vi "Basci_VIs_FindIndexByKeyWords.vi"(4 "error in (no error)":errorcluster, 5 "Max length\nof index":i32=4, 6 "Key words":string="Trace_", 7 "String input":string) -> (0 "error out":errorcluster, 1 "Log":string, 2 "# boundaries between char and digit":i32, 3 "Folder index":i32)   [LabVIEW 2017, in "BasicVIs.lvlib"]
uses:
  BasicVIs.lvlib
panel:
  out "Numeric":i32
  out "Array":u8[](array[numeric])
  out "has digit":bool
  out "has NaN":bool
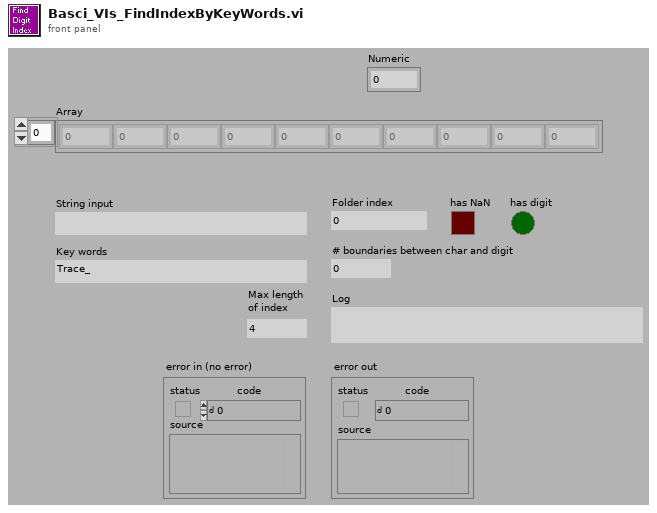
[diagram p1: front panel]
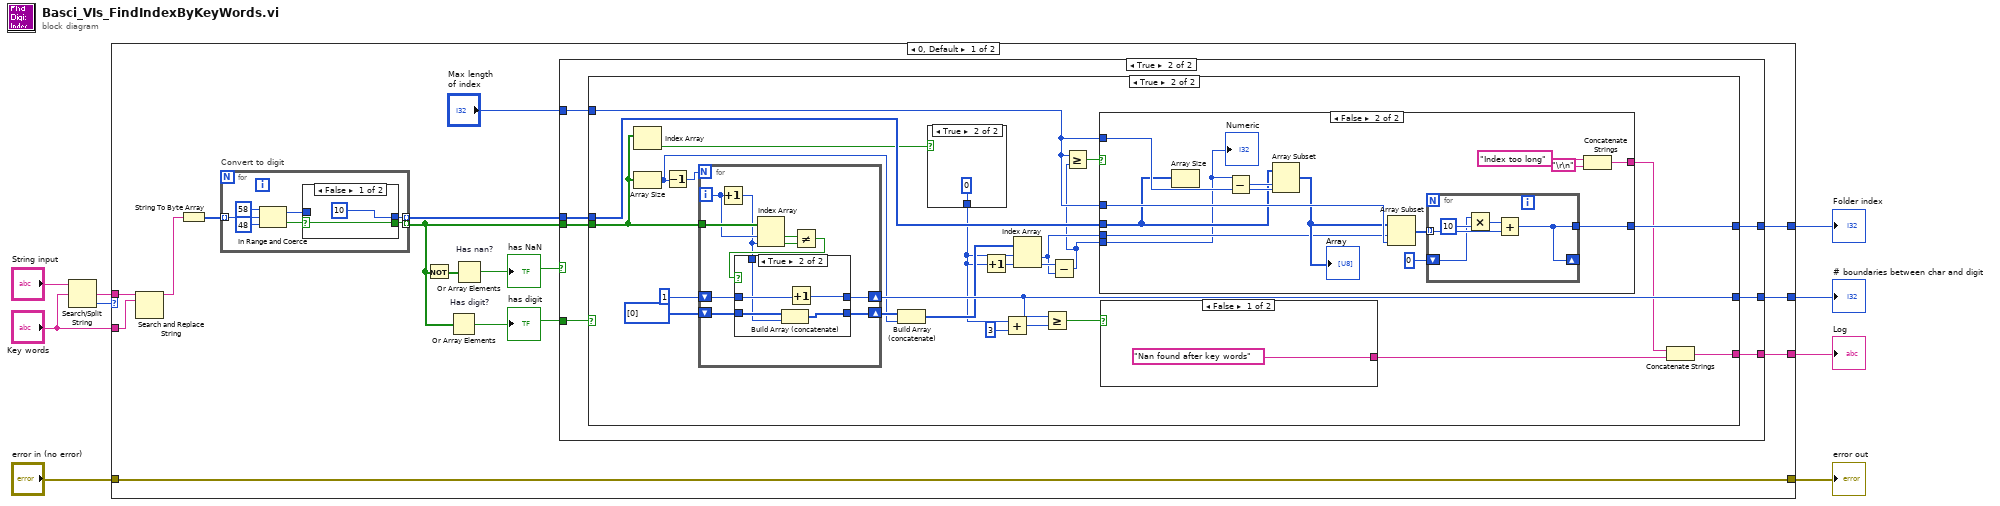
[diagram p0: block diagram]
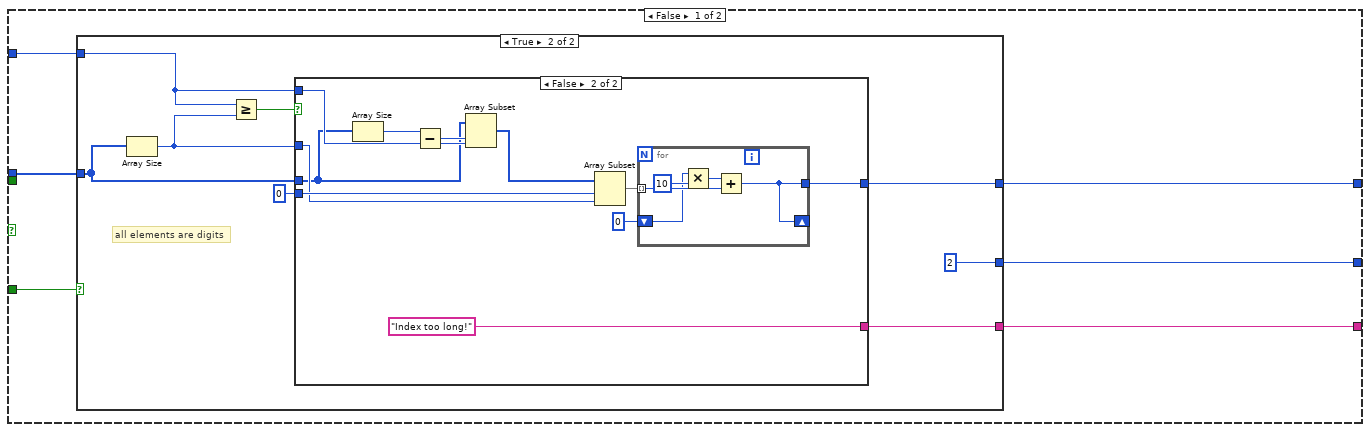
[diagram p2: hidden frame]
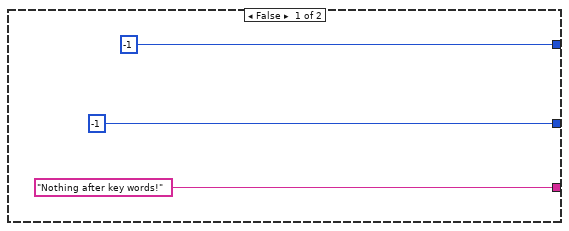
[diagram p3: hidden frame]
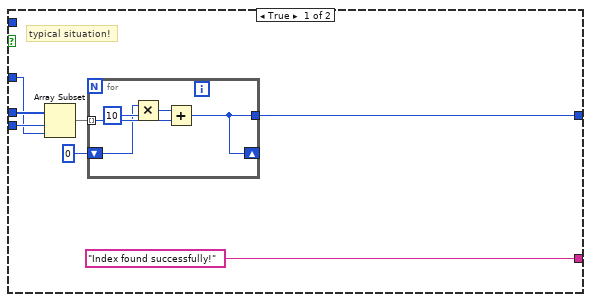
[diagram p4: hidden frame]
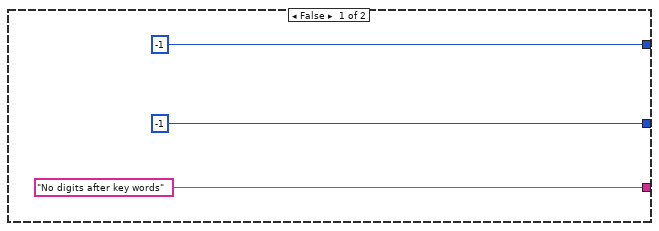
[diagram p5: hidden frame]
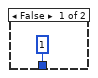
[diagram p6: hidden frame]
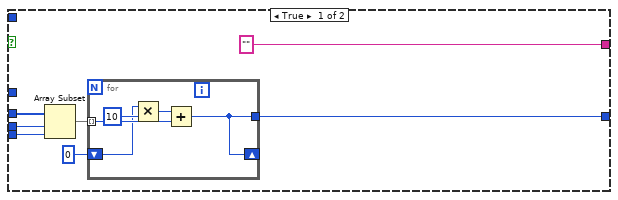
[diagram p7: hidden frame]
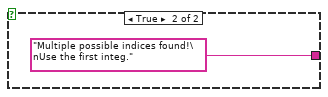
[diagram p8: hidden frame]
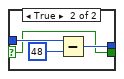
[diagram p10: hidden frame]
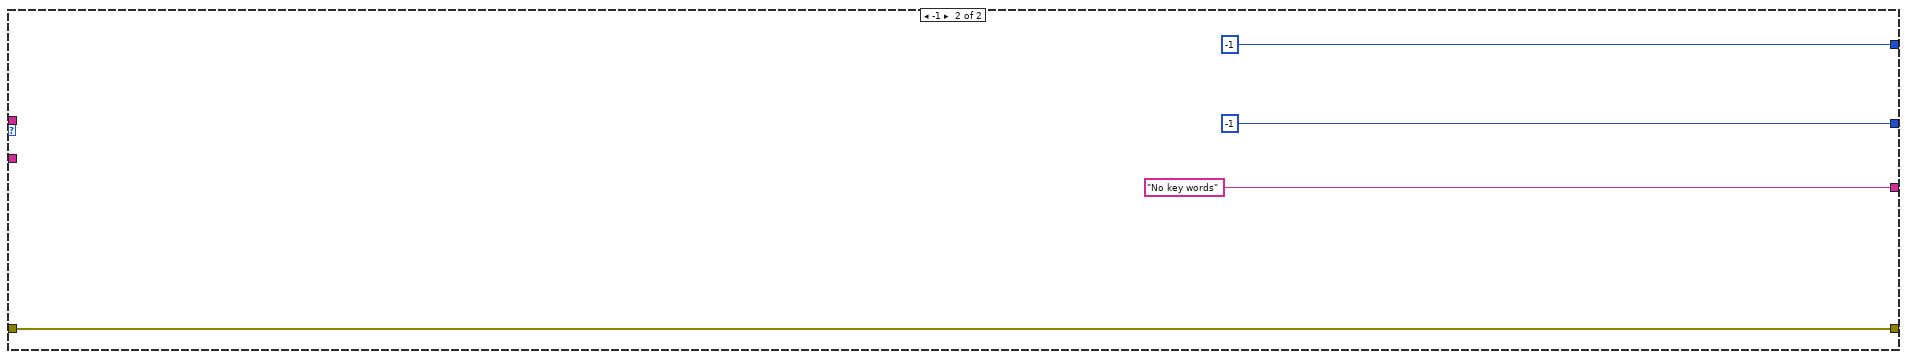
[diagram p11: hidden frame]
diagram:
  n1 = Search/Split String(string="String input", search string/char (-)="Key words") -> (match + rest of string=w8:string, offset of match=w9:i32)  [unwired: 1 in, 1 out]
  n2 = case shown="0, Default" w9 {
    tunnel: w8 -> [w19 _]
    tunnel: [w12 "No key words"] -> w3
    tunnel: "Key words" -> [w18 _]
    tunnel: [w14 -1] -> w4
    tunnel: [w13 -1] -> w5
    tunnel: "error in (no error)" -> [w10 w167]
    tunnel: [w10 w167] -> w1
    frame 0, Default {
      n3 = Search and Replace String(input string=w19, search string=w18) -> (result string=w23:string)  [unwired: 6 in, 3 out]
      n4 = String To Byte Array(string=w23) -> (unsigned byte array=w20:u8[])
      n5 = for "Convert to digit" {
        tunnel: w20 -> [w158] mode=indexing
        tunnel: [w155] -> w17 mode=indexing
        tunnel: [w154] -> w21 mode=indexing
        n6 = In Range and Coerce(upper limit=u8 58, x=w158, lower limit=u8 48) -> (coerced(x)=w157:u8, In Range?=w156:bool)
        n7 = case shown="False" w156 {
          selector: w156 -> [w161 w163]
          tunnel: w157 -> [_ w166]
          tunnel: [u8 10 ("upper limit") w164] -> w154
          tunnel: [w161 w163] -> w155
          frame False {
          }
          frame True {
            n8 = Subtract(x=w166, y=u8 48) -> (x-y=w164:u8)
          }
        }
      }
      n9 = Not(x=w17) -> (.not. x?=w16:bool[])
      n10 = Or Array Elements "Has digit?"(Boolean array=w17) -> (logical OR=w22:bool)
      "has digit" <- w22
      n11 = Or Array Elements "Has nan?"(Boolean array=w16) -> (logical OR=w15:bool)
      "has NaN" <- w15
      n12 = case shown="True" w15 {
        tunnel: w21 -> [w29 w73]
        tunnel: [w28 w72] -> w13
        tunnel: w22 -> [w27 w70]
        tunnel: w17 -> [_ w75]
        tunnel: [w26 w74] -> w14
        tunnel: [w25 w71] -> w12
        tunnel: "Max length\nof index" -> [w24 w69]
        frame False {
          n13 = case shown="True" w27 {
            tunnel: w29 -> [_ w38]
            tunnel: [-1 w34] -> w28
            tunnel: ["Nothing after key words!" w35] -> w25
            tunnel: [-1 2] -> w26
            tunnel: w24 -> [_ w33]
            frame False {
            }
            frame True {
              # "all elements are digits"
              n14 = Array Size(array=w38) -> (size(s)=w36:i32)
              n15 = Greater Or Equal?(x=w33, y=w36) -> (x >= y?=w37:bool)
              n16 = case shown="False" w37 {
                tunnel: 0 -> [w47 w63]
                tunnel: w38 -> [w46 w55]
                tunnel: [w44 w59] -> w34
                tunnel: ["Index found successfully!" "Index too long!"] -> w35
                tunnel: w36 -> [w43 w61]
                tunnel: w33 -> [_ w56]
                frame True {
                  # "typical situation!"
                  n17 = Array Subset(array=w46, index=w47, length=w43) -> (w45:u8[])
                  n18 = for {
                    tunnel: w45 -> [w50] mode=indexing
                    tunnel: [w49] -> w44
                    shift-right: [w49] -> _
                    shift-left: 0 -> [w48]
                    n19 = Multiply(x=w48, y=10) -> (x*y=w51:i32)
                    n20 = Add(x=w51, y=w50) -> (x+y=w49:i32)
                  }
                }
                frame False {
                  n21 = Array Size(array=w55) -> (size(s)=w53:i32)
                  n22 = Subtract(x=w53, y=w56) -> (x-y=w57:i32)
                  n23 = Array Subset(array=w55, index=w57, length=w56) -> (w54:u8[])
                  n24 = Array Subset(array=w54, index=w63, length=w61) -> (w58:u8[])
                  n25 = for {
                    tunnel: w58 -> [w66] mode=indexing
                    tunnel: [w65] -> w59
                    shift-right: [w65] -> _
                    shift-left: 0 -> [w64]
                    n26 = Multiply(x=w64, y=10) -> (x*y=w67:i32)
                    n27 = Add(x=w67, y=w66) -> (x+y=w65:i32)
                  }
                }
              }
            }
          }
        }
        frame True {
          n28 = case shown="True" w70 {
            tunnel: w75 -> [_ w100]
            tunnel: [-1 w99] -> w74
            tunnel: w73 -> [_ w95]
            tunnel: [-1 w94] -> w72
            tunnel: ["No digits after key words" w93] -> w71
            tunnel: w69 -> [_ w92]
            frame False {
            }
            frame True {
              n29 = Index Array(array=w100) -> (element=w79:bool)  [unwired: 1 in]
              n30 = Array Size(array=w100) -> (size(s)=w96:i32)
              n31 = Decrement(x=w96) -> (x-1=w102:i32)
              n32 = for {
                N: w102 -> [_]
                tunnel: w100 -> [w146]
                shift-right: [w140] -> w99
                shift-left: 1 -> [w141]
                shift-right: [w138] -> w98
                shift-left: i32[] [0] -> [w139]
                i -> [w143]
                n33 = Increment(x=w143) -> (x+1=w137:i32)
                n34 = Index Array(array=w146, index #1=w143, index #2=w137) -> (element #1=w145:bool, element #2=w144:bool)
                n35 = Not Equal?(x=w145, y=w144) -> (x != y?=w142:bool)
                n36 = case shown="True" w142 {
                  tunnel: w141 -> [w148 w153]
                  tunnel: [w148 w152] -> w140
                  tunnel: w139 -> [w147 w150]
                  tunnel: [w147 w151] -> w138
                  tunnel: w137 -> [_ w149]
                  frame False {
                  }
                  frame True {
                    n37 = Build Array (concatenate)(w150, w149) -> (w151:i32[])
                    n38 = Increment(x=w153) -> (x+1=w152:i32)
                  }
                }
              }
              n39 = Build Array (concatenate)(w98, w96) -> (w97:i32[])
              n40 = case shown="True" w79 {
                tunnel: [1 ("index") 0 ("index")] -> w86
                frame False {
                }
                frame True {
                }
              }
              n41 = Increment(x=w86) -> (x+1=w87:i32)
              n42 = Add(x=w86, y=3) -> (x+y=w84:i32)
              n43 = Index Array(array=w97, index #1=w86, index #2=w87) -> (element #1=w89:i32, element #2=w90:i32)
              n44 = Greater Or Equal?(x=w99, y=w84) -> (x >= y?=w88:bool)
              n45 = Subtract(x=w90, y=w89) -> (x-y=w82:i32)
              n46 = Greater Or Equal?(x=w92, y=w82) -> (x >= y?=w83:bool)
              n47 = case shown="False" w83 {
                tunnel: w82 -> [w111 w117]
                tunnel: w89 -> [w110 w118]
                tunnel: w95 -> [w109 w120]
                tunnel: [w106 w124] -> w94
                tunnel: w92 -> [_ w129]
                tunnel: ["" w128] -> w80
                tunnel: w92 -> [_ w121]
                frame True {
                  n48 = Array Subset(array=w109, index=w110, length=w111) -> (w105:u8[])
                  n49 = for {
                    tunnel: w105 -> [w114] mode=indexing
                    tunnel: [w113] -> w106
                    shift-right: [w113] -> _
                    shift-left: 0 -> [w112]
                    n50 = Multiply(x=w112, y=10) -> (x*y=w115:i32)
                    n51 = Add(x=w115, y=w114) -> (x+y=w113:i32)
                  }
                }
                frame False {
                  n52 = Array Size(array=w120) -> ()  [unwired: 1 out]
                  n53 = Subtract(x=w117, y=w121) -> (x-y=w122:i32)
                  n54 = Array Subset(array=w120, index=w122, length=w121) -> (w119:u8[])
                  "Array" <- w119
                  n55 = Array Subset(array=w119, index=w118, length=w129) -> (w123:u8[])
                  n56 = for {
                    tunnel: w123 -> [w132] mode=indexing
                    tunnel: [w131] -> w124
                    shift-right: [w131] -> _
                    shift-left: 0 -> [w130]
                    n57 = Multiply(x=w130, y=10) -> (x*y=w133:i32)
                    n58 = Add(x=w133, y=w132) -> (x+y=w131:i32)
                  }
                  n59 = Concatenate Strings("Index too long", "\r\n") -> (w128:string)
                  "Numeric" <- w117
                }
              }
              n60 = case shown="False" w88 {
                tunnel: ["Nan found after key words" "Multiple possible indices found!\nUse the first integ."] -> w81
                frame False {
                }
                frame True {
                }
              }
              n61 = Concatenate Strings(w80, w81) -> (w93:string)
            }
          }
        }
      }
    }
    frame -1 {
    }
  }
  "error out" <- w1
  "Folder index" <- w5
  "# boundaries between char and digit" <- w4
  "Log" <- w3
